vi "Testing For Vision.vi"() -> ()   [LabVIEW 2017]
uses:
  <vilib>/userdefined/High Color/IMAQdx.ctl
  <vilib>/vision/driver/NI_Vision_Acquisition_Software.lvlib
  <vilib>/vision/NI_Vision_Development_Module.lvlib
panel:
  out "error out 3":errorcluster
  out "QR Data":string
  out "error out 5":errorcluster
  out "Data 2":string
  in  "Barcode Types To Search 2":u32[](array[ring])=[6, 4] items=["Reserved", "Codabar", "Code 39", "Code 93", "Code 128", "EAN 8", "EAN 13", "Interleaved 2 of 5", "MSI", "UPCA", "Pharmacode", "RSS Limited"]
  out "error out 4":errorcluster
  in  "Select Vision System":string(combo)="None"
  out "error out 8":errorcluster
  out "error out 2":errorcluster
  out "Image":T1(plugin-control)
  in  "stop":bool
  out "Found":bool
  in  "Session In":T2
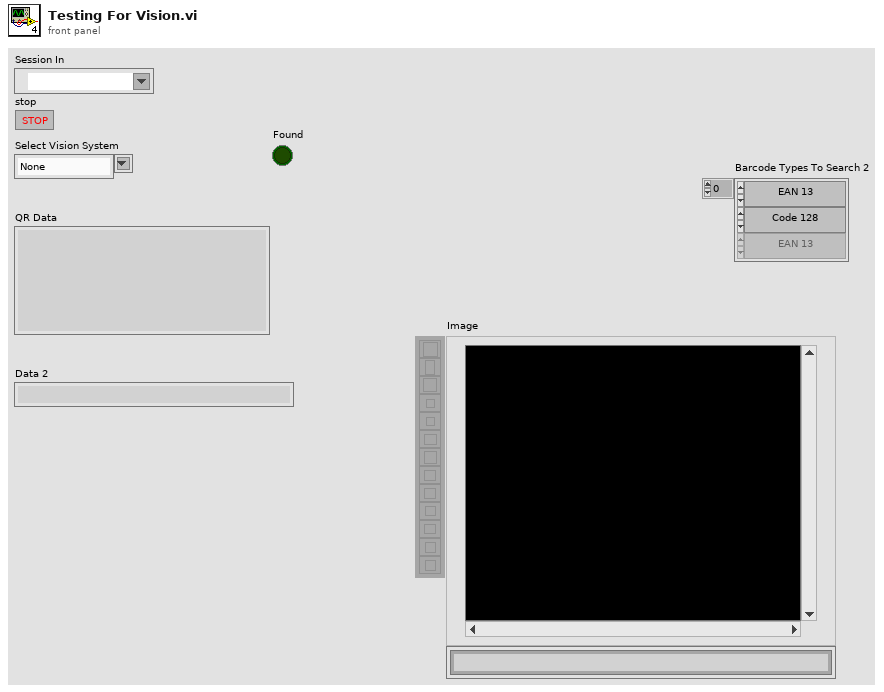
[diagram p1: front panel]
types:
  T1 = typedef "IMAQ Image.ctl" = refnum<image>
  T2 = typedef "IMAQdx.ctl" = refnum<k21>
  T3 = typedef "Image Type" = u32
  T4 = cluster{"Data":string, "Special Char 1":string, "Special Char 2":string, "Checksum(s)":string, "Barcode Type":u32, "Confidence Level":sgl, "Bounding Box":cluster{"x":sgl, "y":sgl}[]}[]
  T5 = cluster{"Data":string, "Special Char 1":string, "Special Char 2":string, "Checksum(s)":string, "Barcode Type":u32, "Confidence Level":sgl, "Bounding Box":cluster{"x":sgl, "y":sgl}[]}
  T6 = typedef "QR Code Report.ctl" = cluster{"Found?":bool, "Data":string, "Bounding Box":cluster{"x":sgl, "y":sgl}[], "Errors Corrected":u32, "Dimensions (Rows/Cols)":u32, "Version":u32, "QR Model":T7, "Stream Mode":T8, "Barcode Polarity":T9, "Mirrored?":bool, "Append Stream Position":u32, "Size of Append Stream":u32, "First EAN-128 ID":i32, "First Alternate Language ID":i32, "Append Stream ID":u32, "Minimum Edge Strength":u32, "Demodulation Mode":T10, "Cell Sample Size":T11, "Cell Filter Mode":T12}
  T7 = typedef "QR Code Model Type.ctl" = i32
  T8 = typedef "QR Code Stream Mode Type.ctl" = i32
  T9 = typedef "Data Matrix Polarity.ctl" = i32
  T10 = typedef "Demodulation Mode.ctl" = i32
  T11 = typedef "Cell Sample Size.ctl" = i32
  T12 = typedef "Cell Filter Mode.ctl" = i32
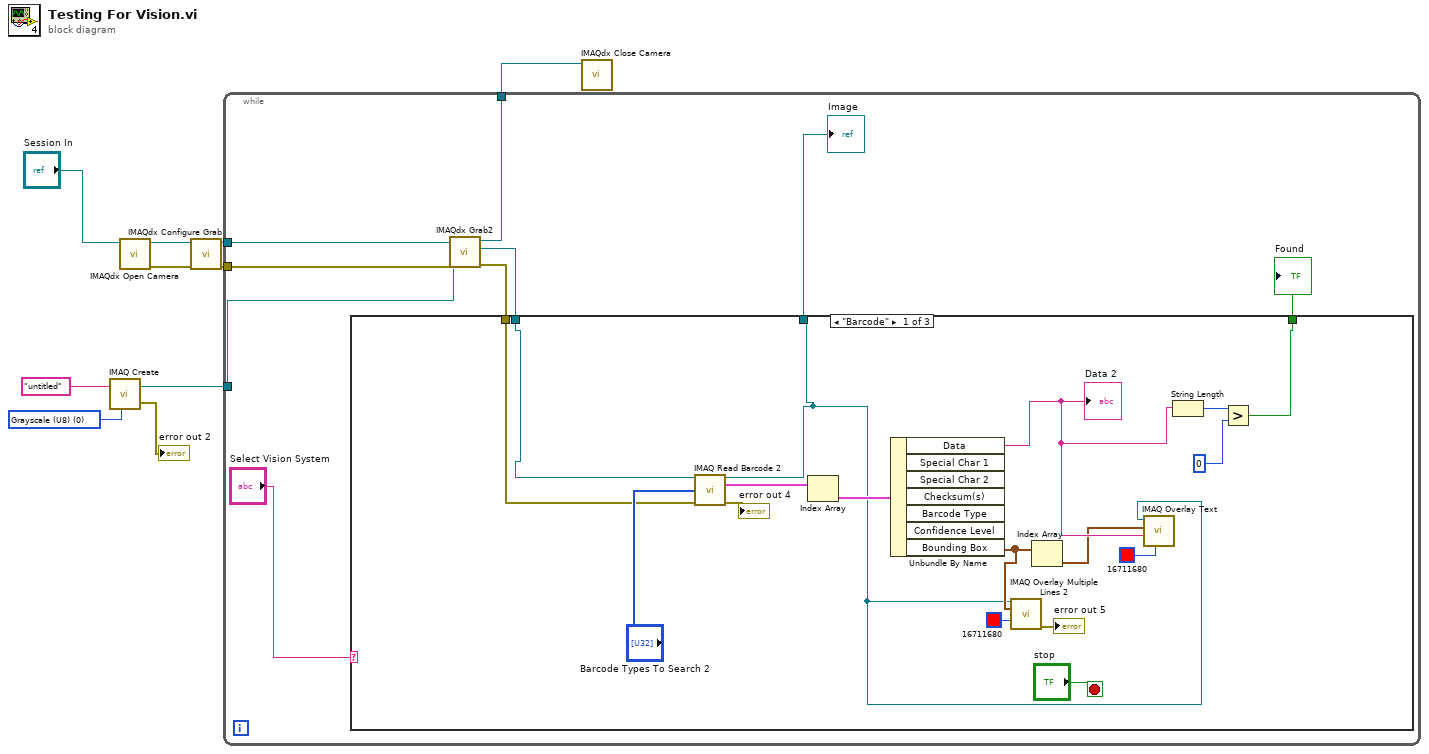
[diagram p0: block diagram]
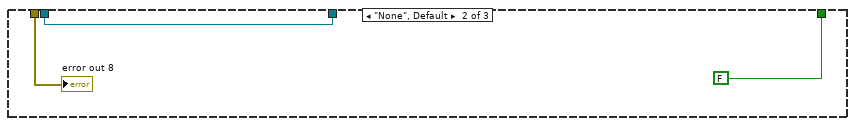
[diagram p2: hidden frame]
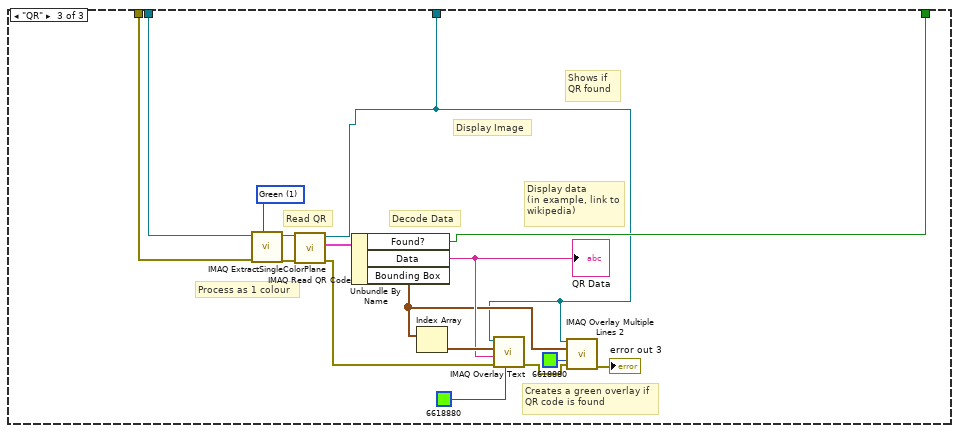
[diagram p3: hidden frame]
diagram:
  w2 = T3 0 items=["Grayscale (U8)", "Grayscale (I16)", "Grayscale (SGL)", "Complex (CSG)", "RGB (U32)", "HSL (U32)", "RGB (U64)", "Grayscale (U16)"] ("Image Type")
  n1 = call "IMAQ Create"("Image Name"="untitled", "Image Type"=w2) -> ("New Image"=w3:T1, "error out"=→"error out 2":errorcluster)  [unwired: 3 in]
  n2 = call <vilib>:"IMAQdx Open Camera.vi"("Session In"="Session In") -> ("error out"=w9:errorcluster, "Session Out"=w10:T2)  [unwired: 9 in]
  n3 = call <vilib>:"IMAQdx Configure Grab.vi"("error in"=w9, "Session In"=w10) -> ("error out"=w4:errorcluster, "Session Out"=w6:T2)  [unwired: 8 in]
  n4 = while {
    tunnel: w6 -> [w20]
    tunnel: [w19] -> w5
    tunnel: w4 -> [w18]
    tunnel: w3 -> [w17]
    stop <- "stop" stop-if-true
    n5 = call <vilib>:"IMAQdx Grab2.vi"("error in"=w18, "Image In"=w17, "Session In"=w20) -> ("error out"=w11:errorcluster, "Image Out"=w15:T1, "Session Out"=w19:T2)  [unwired: 5 in, 1 out]
    n6 = case shown="\"Barcode\"" "Select Vision System" {
      tunnel: w15 -> [w23 w38 w41]
      tunnel: w11 -> [w22 w39 w40]
      tunnel: [w21 FALSE w43] -> w14
      tunnel: [w24 w38 w42] -> w13
      frame "Barcode" {
        n7 = call "IMAQ Read Barcode 2"("Image"=w23, "Barcode Types To Search"="Barcode Types To Search 2", "error in (no error)"=w22) -> ("Image (duplicate)"=w24:T1, "Barcodes"=w30:T4, "error out"=→"error out 4":errorcluster)  [unwired: 8 in, 2 out]
        n8 = Index Array(array=w30) -> (element=w31:T5)  [unwired: 1 in]
        n9 = Unbundle By Name(w31) -> ("Data"=w35:string, "Bounding Box"=w33:cluster{"x":sgl, "y":sgl}[])  [unwired: 5 out]
        "Data 2" <- w35
        n10 = call "IMAQ Overlay Multiple Lines 2"("Image"=w24, "Line End Points"=w33, "Color"=u32 16711680) -> ("error out"=→"error out 5":errorcluster)  [unwired: 11 in, 1 out]
        n11 = Index Array(array=w33) -> (element=w32:cluster{"x":sgl, "y":sgl})  [unwired: 1 in]
        n12 = call "IMAQ Overlay Text"("Text Color (black)"=u32 16711680, "String"=w35, "Origin"=w32, "Image"=w24) -> ()  [unwired: 6 in, 2 out]
        n13 = String Length(string=w35) -> (length=w36:i32)
        n14 = Greater?(x=w36, y=0) -> (0:w21:bool)
      }
      frame "None", Default {
        "error out 8" <- w39
      }
      frame "QR" {
        w53 = 1 items=["Red", "Green", "Blue", "Hue", "Saturation", "Luminance", "Value", "Intensity"] ("Color Plane")
        # "Creates a green overlay if\nQR code is found"
        # "Shows if\nQR found"
        # "Display data\n(in example, link to wikipedia)"
        # "Decode Data"
        # "Display Image"
        # "Read QR"
        # "Process as 1 colour"
        n15 = call "IMAQ ExtractSingleColorPlane"("Color Plane"=w53, "error in (no error)"=w40, "Image Src"=w41) -> ("error out"=w54:errorcluster, "Image Dst Out"=w55:T1)  [unwired: 7 in]
        n16 = call "IMAQ Read QR Code"("error in (no error)"=w54, "Image"=w55) -> ("error out"=w44:errorcluster, "QR Code Report"=w52:T6, "Image (duplicate)"=w42:T1)  [unwired: 6 in, 1 out]
        n17 = Unbundle By Name(w52) -> ("Found?"=w43:bool, "Data"=w50:string, "Bounding Box"=w48:cluster{"x":sgl, "y":sgl}[])
        "QR Data" <- w50
        n18 = Index Array(array=w48) -> (element=w51:cluster{"x":sgl, "y":sgl})  [unwired: 1 in]
        n19 = call "IMAQ Overlay Text"("Text Color (black)"=u32 6618880, "error in (no error)"=w44, "String"=w50, "Origin"=w51, "Image"=w42) -> ("error out"=w46:errorcluster)  [unwired: 5 in, 1 out]
        n20 = call "IMAQ Overlay Multiple Lines 2"("Image"=w42, "Line End Points"=w48, "Color"=u32 6618880, "error in (no error)"=w46) -> ("error out"=→"error out 3":errorcluster)  [unwired: 10 in, 1 out]
      }
    }
    "Image" <- w13
    "Found" <- w14
  }
  n21 = call <vilib>:"IMAQdx Close Camera.vi"("Session In"=w5) -> ()  [unwired: 10 in, 1 out]
